vi "36_Water Level Checker.vi"() -> ()   [LabVIEW 2022 SP3]
panel:
  out "Water Level is Low":bool
  out "Water Level is High":bool
  out "Water Level":u8(slide) scale=0.0..10.0
  in  "Water Tanker":dbl(slide) scale=0.0..10.0
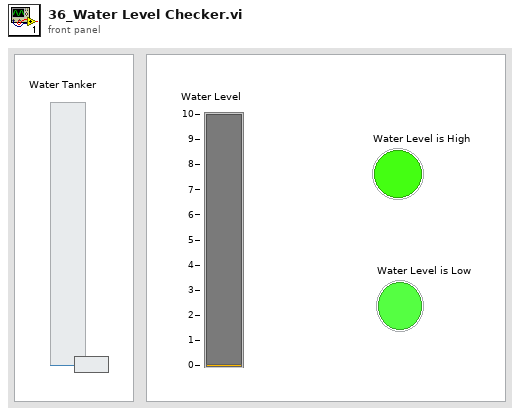
[diagram p1: front panel]
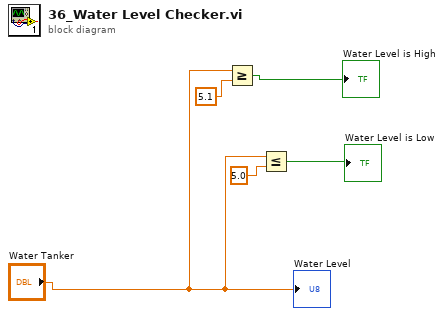
[diagram p0: block diagram]
diagram:
  n1 = Greater Or Equal?(x="Water Tanker", y=5.1) -> (x >= y?=→"Water Level is High":bool)
  n2 = Less Or Equal?(x="Water Tanker", y=5.0) -> (x <= y?=→"Water Level is Low":bool)
  "Water Level" <- "Water Tanker"
